vi "LoopAddShiftRegister.vi"(0 "__args":T1) -> (2 "__errStatus":bool, 3 "__errCode":i32, 4 "__errSource":string)   [LabVIEW 2013]
panel:
  out "__return":i32[](array[numeric])
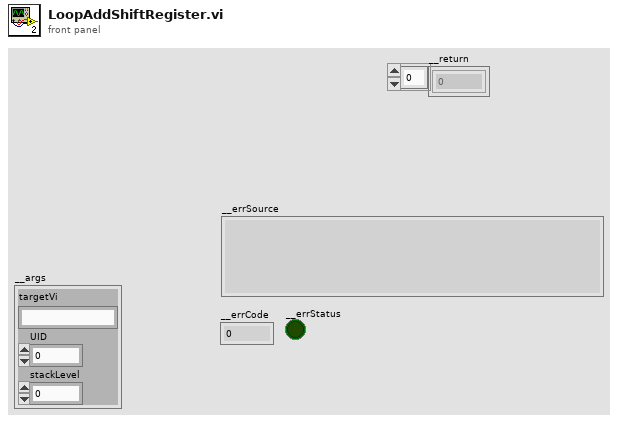
[diagram p1: front panel]
types:
  T1 = cluster{"targetVi":string, "UID":i32, "stackLevel":i32}
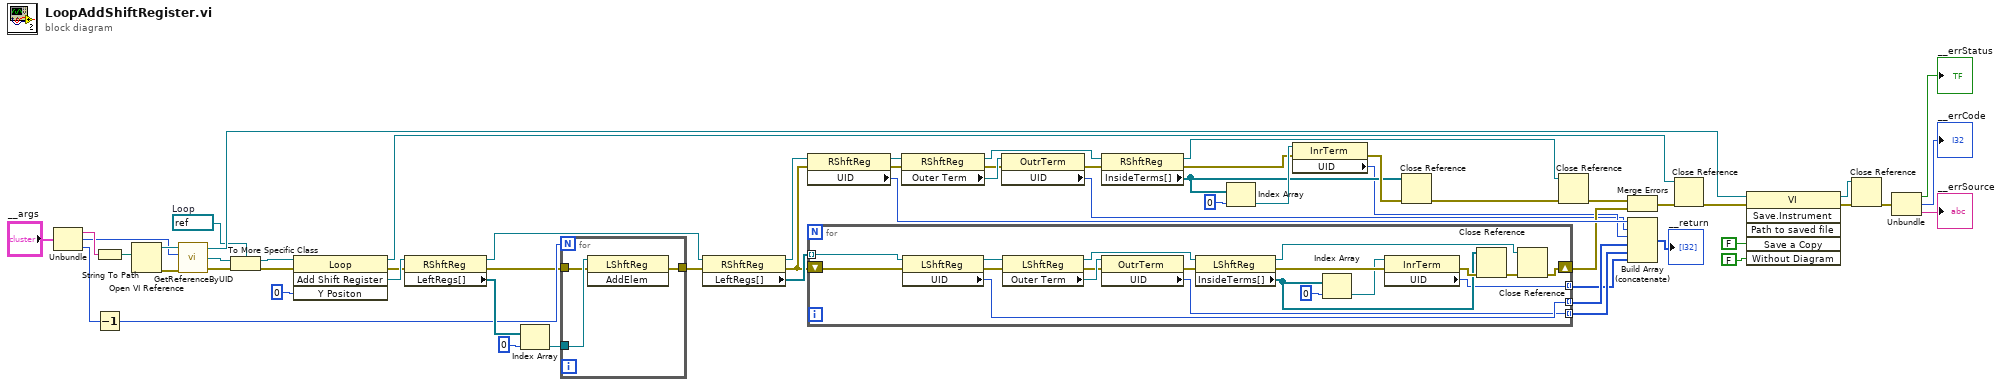
[diagram p0: block diagram]
diagram:
  w42 = refnum<vi> refnum  # Loop
  n1 = Unbundle("__args") -> ("targetVi"=w53:string, "UID"=w38:i32, "stackLevel"=w32:i32)
  n2 = String To Path(string=w53) -> (path=w55:path)
  n3 = Decrement(x=w32) -> (x-1=w33:i32)
  n4 = Open VI Reference(vi path=w55) -> (vi reference=w52:refnum<vi>, error out=w54:errorcluster)  [unwired: 5 in]
  n5 = call "GetReferenceByUID.vi"("error in (no error)"=w54, "UID"=w38, "targetVI"=w52) -> ("error out"=w51:errorcluster, "refNum"=w50:refnum<vi>, "dup targetVI"=w46:refnum<vi>)  [unwired: 1 in]
  n6 = To More Specific Class(target class=w42, reference=w50, error in=w51) -> (specific class reference=w41:refnum<vi>, error out=w40:errorcluster)
  n7 = invoke class="Loop" method="Add Shift Register"(reference=w41, error in=w40, "Y Positon"=u32 0) -> (reference out=w39:refnum<vi>, error out=w31:errorcluster, "Add Shift Register"=w37:refnum<vi>)  [unwired: 1 in, 1 out]
  n8 = property class="RShftReg"(reference=w37, error in=w31) -> (reference out=w29:refnum<vi>, error out=w30:errorcluster, "LeftRegs[]"=w36:refnum<vi>[])
  n9 = Index Array(array=w36, index=0) -> (element=w34:refnum<vi>)
  n10 = for {
    N: w33 -> [_]
    tunnel: w34 -> [w62]
    tunnel: w30 -> [w61]
    tunnel: [w60] -> w28
    n11 = invoke class="LShftReg" method="AddElem"(reference=w62, error in=w61) -> (error out=w60:errorcluster)  [unwired: 1 in, 2 out]
  }
  n12 = property class="RShftReg"(reference=w29, error in=w28) -> (reference out=w27:refnum<vi>, error out=w20:errorcluster, "LeftRegs[]"=w25:refnum<vi>[])
  n13 = property class="RShftReg"(reference=w27, error in=w20) -> (reference out=w11:refnum<vi>, error out=w10:errorcluster, "UID"=w22:i32)
  n14 = for {
    tunnel: w25 -> [w81] mode=indexing
    shift-right: [w76] -> w19
    shift-left: w20 -> [w77]
    tunnel: [w66] -> w3 mode=indexing
    tunnel: [w65] -> w2 mode=indexing
    tunnel: [w64] -> w1 mode=indexing
    n15 = property class="LShftReg"(reference=w81, error in=w77) -> (reference out=w67:refnum<vi>, error out=w69:errorcluster, "UID"=w66:i32)
    n16 = property class="LShftReg"(reference=w67, error in=w69) -> (reference out=w63:refnum<vi>, error out=w70:errorcluster, "Outer Term"=w71:refnum<vi>)
    n17 = property class="OutrTerm"(reference=w71, error in=w70) -> (error out=w68:errorcluster, "UID"=w65:i32)  [unwired: 1 out]
    n18 = property class="LShftReg"(reference=w63, error in=w68) -> (reference out=w72:refnum<vi>, error out=w79:errorcluster, "InsideTerms[]"=w73:refnum<vi>[])
    n19 = Index Array(array=w73, index=0) -> (element=w78:refnum<vi>)
    n20 = property class="InrTerm"(reference=w78, error in=w79) -> (error out=w74:errorcluster, "UID"=w64:i32)  [unwired: 1 out]
    n21 = Close Reference(reference=w73, error in (no error)=w74) -> (error out=w75:errorcluster)
    n22 = Close Reference(reference=w72, error in (no error)=w75) -> (error out=w76:errorcluster)
  }
  n23 = property class="RShftReg"(reference=w11, error in=w10) -> (reference out=w9:refnum<vi>, error out=w7:errorcluster, "Outer Term"=w8:refnum<vi>)
  n24 = property class="OutrTerm"(reference=w8, error in=w7) -> (error out=w6:errorcluster, "UID"=w4:i32)  [unwired: 1 out]
  n25 = property class="RShftReg"(reference=w9, error in=w6) -> (reference out=w13:refnum<vi>, error out=w23:errorcluster, "InsideTerms[]"=w14:refnum<vi>[])
  n26 = Index Array(array=w14, index=0) -> (element=w24:refnum<vi>)
  n27 = property class="InrTerm"(reference=w24, error in=w23) -> (error out=w15:errorcluster, "UID"=w5:i32)  [unwired: 1 out]
  n28 = Close Reference(reference=w14, error in (no error)=w15) -> (error out=w17:errorcluster)
  n29 = Close Reference(reference=w13, error in (no error)=w17) -> (error out=w16:errorcluster)
  n30 = Merge Errors(w16, w19) -> (w18:errorcluster)
  n31 = Build Array (concatenate)(w22, w4, w5, w3, w2, w1) -> (→"__return":i32[])
  n32 = Close Reference(reference=w39, error in (no error)=w18) -> (error out=w45:errorcluster)
  n33 = invoke class="VI" method="Save.Instrument"(reference=w46, error in=w45, "Save a Copy"=FALSE, "Without Diagram"=FALSE) -> (reference out=w43:refnum<vi>, error out=w44:errorcluster)  [unwired: 2 in, 4 out]
  n34 = Close Reference(reference=w43, error in (no error)=w44) -> (error out=w49:errorcluster)
  n35 = Unbundle(w49) -> ("status"=→"__errStatus":bool, "code"=→"__errCode":i32, "source"=→"__errSource":string)
